vi "Is Even.vi"(1 "Element":i32) -> (0 "Value":bool)   [LabVIEW 2020, in "Examples.lvlib"]
uses:
  Examples.lvlib
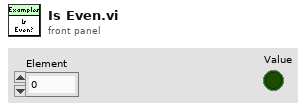
[diagram p1: front panel]
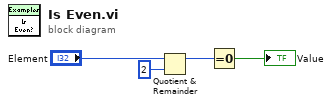
[diagram p0: block diagram]
diagram:
  n1 = Quotient & Remainder(x="Element", y=2) -> (x-y*floor(x/y)=w3:i32)  [unwired: 1 out]
  n2 = Equal To 0?(x=w3) -> (x = 0?=→"Value":bool)
